vi "FeedbackDecode.vi"() -> ()   [LabVIEW 2020]
uses:
  FeedbackDecode_DecodeClust.ctl
  FeedbackDecode_MvntClust.ctl
  FeedbackDecode_EncodeClust.ctl
  FeedbackDecode_CogLoadClust.ctl
  <vilib>/Platform/TimedLoop/XDataNode/timing_clust.ctl
  <vilib>/Platform/TimedLoop/XDataNode/nitl_modes.ctl
  <vilib>/Platform/TimedLoop/XDataNode/wakeup.ctl
  <vilib>/DAQmx/write.llb/DAQmx Write (Analog DBL 1Chan 1Samp).vi
  subvi/FeedbackDecode_Globals.vi
  <vilib>/imath/engines/lvmath2/RunTimeEngine/BuiltInFunctions/reshapemx/NIMS_[GM]_reshapemx.vi
  <instcachedir>/0/NIMS_[GM]_reshapemx_98F4FEDA5D2741A4824CEDFB6097FB68.lvgen/NIMS_[GM]_reshapemx_98F4FEDA5D2741A4824CEDFB6097FB68_005.vi
  <vilib>/imath/engines/lvmath2/RunTimeEngine/BuiltInFunctions/rotate90/NIMS_rotate90.vi
  <instcachedir>/0/NIMS_rotate90_7DC1660D109944E092D2EB6E3185A1B6.lvgen/NIMS_rotate90_7DC1660D109944E092D2EB6E3185A1B6_005.vi
  <vilib>/imath/engines/lvmath2/RunTimeEngine/BuiltInFunctions/reshapemx/NIMS_[GV]_reshapemx.vi
  <instcachedir>/0/NIMS_[GV]_reshapemx_116A7F60707440F78CB0D64335A3F73C.lvgen/NIMS_[GV]_reshapemx_116A7F60707440F78CB0D64335A3F73C_001.vi
  <vilib>/imath/engines/lvmath2/RunTimeEngine/ErrorHandling/NIMS_Create Error From Enums.vi
  <vilib>/imath/engines/lvmath2/RunTimeEngine/NodeEndStatement/NIMS_NodeEndStatement_Output.vi
  <instcachedir>/0/NIMS_NodeEndStatement_Output_53EC0D466D134D7ABD903AC30B43404B.lvgen/NIMS_NodeEndStatement_Output_53EC0D466D134D7ABD903AC30B43404B_004.vi
  <vilib>/imath/engines/lvmath2/RunTimeEngine/ErrorHandling/NIMS_Finalize Error.vi
  subvi/FeedbackDecode_VariablesToString_Scalar.vi
  <vilib>/DAQmx/miscellaneous.llb/DAQmx Fill In Error Info.vi
  subvi/FeedbackDecode_VariablesToString_String.vi
  subvi/FeedbackDecode_VariablesToString_Array.vi
  <vilib>/Utility/file.llb/Read Delimited Spreadsheet (string).vi
  <vilib>/Utility/file.llb/Write Delimited Spreadsheet (string).vi
  <vilib>/platform/TimedLoop/XDataNode/XDataNode.xnode
  <vilib>/regexp/Match Regular Expression.xnode
  <vilib>/Platform/TimedLoop/XDataNode/XDNodeRunTimeDep.lvlib
  <resource>/objmgr/daqmx.rc
panel:
  out "ResourcesDir":path=path "Z:/Shared drives/CNI/Tasks/FeedbackDecode/resources"
  out "CurrMvnt":T1={"MvntMat"=[], "MvntName"="", "Tracking"=enum."False", "Radius"=0.15}
  in  "Exclude SE":bool
  out "DAQmx?":bool=TRUE
  out "NumComp":enum16{"1 Computer", "2 Computers"}(ring)
  out "BuildDir":path=path "/\"Z/Shared drives/CNI/Tasks/FeedbackDecode/build\""
  out "PupilTracker":bool
  out "CopySucc":bool
  out "Delete from D drive?":bool
  out "Copy to raid?":bool
  out "Don't save to database?":bool
  out "NextIdx":dbl
  in  "HeatMap Range":cluster{"Min":dbl, "Max":dbl}={"Min"=0.0, "Max"=50.0}
  out "RespRefArray":refnum<vi>[](array[refnum])
  out "VRELabel":T2(ring)
  out "StimTog":bool
  out "SelTog":bool
  out "StimCmd":string
  out "RespStr":string
  out "EvntReg":refnum<event-registration>
  out "MvntEvnt":refnum<user-event>
  out "DataDir":path=path "D:/FeedbackDecode"
  out "PulseStim":bool
  out "BaseCnt3":i64=-9223372036854775808
  out "NIPTime":dbl
  out "ParamsTableLoc":cluster{"Left":i32, "Width":u32}={"Left"=1206, "Width"=743}
  out "iTiming":T3={"Dur"={"ASD"=1000.0, "ARD"=5000.0, "ART"=5000.0, "ETD"=500.0}, "Rnd"={"ASDR"=0.0, "ARDR"=0.0, "ARTR"=0.0, "ETDR"=0.0}, "Act"={"ASDA"=0.0, "ARDA"=0.0, "ARTA"=0.0, "ETDA"=0.0}}
  in  "LVTab":T4(tab)
  out "TrainCnt":dbl
  in  "DecodeClust":T5={"TrainParams"={"Lag"=0.0, "KernelWidth"=0.3, "TargRad"=0.15}, "Kinematics"={"Thumb"=0.0, "Index"=0.0, "Middle"=0.0, "Ring"=0.0, "Little"=0.0, "ThumbInt"=0.0, "IndexInt"=0.0, "RingInt"=0.0, "LittleInt"=0.0, "Wrist"=0.0, "WristYaw"=0.0, "WristRoll"=0.0}, "CtrlButtons"={"AcqTraining"=FALSE, "ApplyBaseline"=FALSE, "ApplyTraining"=FALSE, "LoadTrainFile"=FALSE, "CAR"=FALSE, "NIPSpikes"=FALSE, "AcqBaseline"=FALSE, "Stop"=FALSE, "ResetTrial"=FALSE, "CalDEKA"=FALSE, "HideSphrs"=FALSE, "StartTrials"=FALSE, "AutoPop"=FALSE, "ResetVRE"=FALSE, "StopVRE"=FALSE, "AcqCAR"=FALSE, "ConARD"=FALSE, "DEKARestart"=FALSE, "ConnDEKA"=FALSE}, "CompID"={"LV"={"Name"="PNILABVIEW", "IP"="127.0.0.1"}, "ML"={"Name"="PNIMATLAB", "IP"="127.0.0.2"}}, "KMvntClust"={"KGain"=[[1.0, 1.0, -1.0, 1.0], [1.0, 1.0, -1.0, 1.0], [1.0, 1.0, -1.0, 1.0], [1.0, 1.0, -1.0, 1.0], [1.0, 1.0, -1.0, 1.0], [1.0, 1.0, -1.0, 1.0], [1.0, 1.0, -1.0, 1.0], [1.0, 1.0, -1.0, 1.0], [1.0, 1.0, -1.0, 1.0], [1.0, 1.0, -1.0, 1.0], [1.0, 1.0, -1.0, 1.0], [1.0, 1.0, -1.0, 1.0]], "KMvnts"={"Thumb"=TRUE, "Index"=TRUE, "Middle"=TRUE, "Ring"=TRUE, "Little"=TRUE, "ThumbInt"=TRUE, "IndexInt"=TRUE, "RingInt"=TRUE, "LittleInt"=TRUE, "WristPitch"=TRUE, "WristYaw"=TRUE, "WristRoll"=TRUE}, "KThresh"=[[0.2, 0.2, -1.0, 1.0], [0.2, 0.2, -1.0, 1.0], [0.2, 0.2, -1.0, 1.0], [0.2, 0.2, -1.0, 1.0], [0.2, 0.2, -1.0, 1.0], [0.2, 0.2, -1.0, 1.0], [0.2, 0.2, -1.0, 1.0], [0.2, 0.2, -1.0, 1.0], [0.2, 0.2, -1.0, 1.0], [0.2, 0.2, -1.0, 1.0], [0.2, 0.2, -1.0, 1.0], [0.2, 0.2, -1.0, 1.0]], "CtrlMode"=[enum."Position", enum."Position", enum."Position", enum."Position", enum."Position", enum."Position", enum."Position", enum."Position", enum."Position", enum."Position", enum."Position", enum."Position"], "CtrlSpd"=[1.0, 1.0, 1.0, 1.0, 1.0, 1.0, 1.0, 1.0, 1.0, 1.0, 1.0, 1.0]}, "ClearUEA"=FALSE, "Targets"={"Thumb"=0.0, "Index"=0.0, "Middle"=0.0, "Ring"=0.0, "Little"=0.0, "ThumbInt"=0.0, "IndexInt"=0.0, "RingInt"=0.0, "LittleInt"=0.0, "Wrist"=0.0, "WristYaw"=0.0, "WristRoll"=0.0}, "KUEAArray"=[{"Boolean 1"=FALSE, "Boolean 2"=FALSE, "Boolean 3"=FALSE, "Boolean 4"=FALSE, "Boolean 5"=FALSE, "Boolean 6"=FALSE, "Boolean 7"=FALSE, "Boolean 8"=FALSE, "Boolean 9"=FALSE, "Boolean 10"=FALSE, "Boolean 11"=FALSE, "Boolean 12"=FALSE, "Boolean 13"=FALSE, "Boolean 14"=FALSE, "Boolean 15"=FALSE, "Boolean 16"=FALSE, "Boolean 17"=FALSE, "Boolean 18"=FALSE, "Boolean 19"=FALSE, "Boolean 20"=FALSE, "Boolean 21"=FALSE, "Boolean 22"=FALSE, "Boolean 23"=FALSE, "Boolean 24"=FALSE, "Boolean 25"=FALSE, "Boolean 26"=FALSE, "Boolean 27"=FALSE, "Boolean 28"=FALSE, "Boolean 29"=FALSE, "Boolean 30"=FALSE, "Boolean 31"=FALSE, "Boolean 32"=FALSE, "Boolean 33"=FALSE, "Boolean 34"=FALSE, "Boolean 35"=FALSE, "Boolean 36"=FALSE, "Boolean 37"=FALSE, "Boolean 38"=FALSE, "Boolean 39"=FALSE, "Boolean 40"=FALSE, "Boolean 41"=FALSE, "Boolean 42"=FALSE, "Boolean 43"=FALSE, "Boolean 44"=FALSE, "Boolean 45"=FALSE, "Boolean 46"=FALSE, "Boolean 47"=FALSE, "Boolean 48"=FALSE, "Boolean 49"=FALSE, "Boolean 50"=FALSE, "Boolean 51"=FALSE, "Boolean 52"=FALSE, "Boolean 53"=FALSE, "Boolean 54"=FALSE, "Boolean 55"=FALSE, "Boolean 56"=FALSE, "Boolean 57"=FALSE, "Boolean 58"=FALSE, "Boolean 59"=FALSE, "Boolean 60"=FALSE, "Boolean 61"=FALSE, "Boolean 62"=FALSE, "Boolean 63"=FALSE, "Boolean 64"=FALSE, "Boolean 65"=FALSE, "Boolean 66"=FALSE, "Boolean 67"=FALSE, "Boolean 68"=FALSE, "Boolean 69"=FALSE, "Boolean 70"=FALSE, "Boolean 71"=FALSE, "Boolean 72"=FALSE, "Boolean 73"=FALSE, "Boolean 74"=FALSE, "Boolean 75"=FALSE, "Boolean 76"=FALSE, "Boolean 77"=FALSE, "Boolean 78"=FALSE, "Boolean 79"=FALSE, "Boolean 80"=FALSE, "Boolean 81"=FALSE, "Boolean 82"=FALSE, "Boolean 83"=FALSE, "Boolean 84"=FALSE, "Boolean 85"=FALSE, "Boolean 86"=FALSE, "Boolean 87"=FALSE, "Boolean 88"=FALSE, "Boolean 89"=FALSE, "Boolean 90"=FALSE, "Boolean 91"=FALSE, "Boolean 92"=FALSE, "Boolean 93"=FALSE, "Boolean 94"=FALSE, "Boolean 95"=FALSE, "Boolean 96"=FALSE, "Boolean 97"=FALSE, "Boolean 98"=FALSE, "Boolean 99"=FALSE, "Boolean 100"=FALSE}, {"Boolean 1"=FALSE, "Boolean 2"=FALSE, "Boolean 3"=FALSE, "Boolean 4"=FALSE, "Boolean 5"=FALSE, "Boolean 6"=FALSE, "Boolean 7"=FALSE, "Boolean 8"=FALSE, "Boolean 9"=FALSE, "Boolean 10"=FALSE, "Boolean 11"=FALSE, "Boolean 12"=FALSE, "Boolean 13"=FALSE, "Boolean 14"=FALSE, "Boolean 15"=FALSE, "Boolean 16"=FALSE, "Boolean 17"=FALSE, "Boolean 18"=FALSE, "Boolean 19"=FALSE, "Boolean 20"=FALSE, "Boolean 21"=FALSE, "Boolean 22"=FALSE, "Boolean 23"=FALSE, "Boolean 24"=FALSE, "Boolean 25"=FALSE, "Boolean 26"=FALSE, "Boolean 27"=FALSE, "Boolean 28"=FALSE, "Boolean 29"=FALSE, "Boolean 30"=FALSE, "Boolean 31"=FALSE, "Boolean 32"=FALSE, "Boolean 33"=FALSE, "Boolean 34"=FALSE, "Boolean 35"=FALSE, "Boolean 36"=FALSE, "Boolean 37"=FALSE, "Boolean 38"=FALSE, "Boolean 39"=FALSE, "Boolean 40"=FALSE, "Boolean 41"=FALSE, "Boolean 42"=FALSE, "Boolean 43"=FALSE, "Boolean 44"=FALSE, "Boolean 45"=FALSE, "Boolean 46"=FALSE, "Boolean 47"=FALSE, "Boolean 48"=FALSE, "Boolean 49"=FALSE, "Boolean 50"=FALSE, "Boolean 51"=FALSE, "Boolean 52"=FALSE, "Boolean 53"=FALSE, "Boolean 54"=FALSE, "Boolean 55"=FALSE, "Boolean 56"=FALSE, "Boolean 57"=FALSE, "Boolean 58"=FALSE, "Boolean 59"=FALSE, "Boolean 60"=FALSE, "Boolean 61"=FALSE, "Boolean 62"=FALSE, "Boolean 63"=FALSE, "Boolean 64"=FALSE, "Boolean 65"=FALSE, "Boolean 66"=FALSE, "Boolean 67"=FALSE, "Boolean 68"=FALSE, "Boolean 69"=FALSE, "Boolean 70"=FALSE, "Boolean 71"=FALSE, "Boolean 72"=FALSE, "Boolean 73"=FALSE, "Boolean 74"=FALSE, "Boolean 75"=FALSE, "Boolean 76"=FALSE, "Boolean 77"=FALSE, "Boolean 78"=FALSE, "Boolean 79"=FALSE, "Boolean 80"=FALSE, "Boolean 81"=FALSE, "Boolean 82"=FALSE, "Boolean 83"=FALSE, "Boolean 84"=FALSE, "Boolean 85"=FALSE, "Boolean 86"=FALSE, "Boolean 87"=FALSE, "Boolean 88"=FALSE, "Boolean 89"=FALSE, "Boolean 90"=FALSE, "Boolean 91"=FALSE, "Boolean 92"=FALSE, "Boolean 93"=FALSE, "Boolean 94"=FALSE, "Boolean 95"=FALSE, "Boolean 96"=FALSE, "Boolean 97"=FALSE, "Boolean 98"=FALSE, "Boolean 99"=FALSE, "Boolean 100"=FALSE}], "ReTrain"=FALSE, "TargDist"=[0.0, 0.0, 0.0, 0.0, 0.0, 0.0], "State"=enum."Initialize", "KalmanType"=enum."Mean", "EventStr"="SS.KalmanElects=[];SS.KalmanMvnts=[1,2,3,4,5,6,7,8,9,10,11,12];SS.KalmanGain=[1.0,1.0;1.0,1.0;1.0,1.0;1.0,1.0;1.0,1.0;1.0,1.0;1.0,1.0;1.0,1.0;1.0,1.0;1.0,1.0;1.0,1.0;1.0,1.0;];SS.KalmanThresh=[0.2,0.2;0.2,0.2;0.2,0.2;0.2,0.2;0.2,0.2;0.2,0.2;0.2,0.2;0.2,0.2;0.2,0.2;0.2,0.2;0.2,0.2;0.2,0.2;];SS.CtrlMode={'Position','Position','Position','Position','Position','Position','Position','Position','Position','Position','Position','Position'};SS.CtrlSpeed=[1.0,1.0,1.0,1.0,1.0,1.0,1.0,1.0,1.0,1.0,1.0,1.0];SS.Lag=0.00;SS.KernelWidth=0.30;SS.TargRad=0.15;SS.DataFolder='20210325-092059';SS.DataDir='D@\\FeedbackDecode';SS.BuildDir='Z@\\Shared drives\\CNI\\Tasks\\FeedbackDecode\\build';SS.BadUEAElects=[];SS.SelElect=0;SS.ThreshMode='RMS Auto';SS.ThreshVal=-5.00;SS.AcqTraining=0;SS.ApplyBaseline=0;SS.ApplyTraining=0;SS.LoadTrainFile=0;SS.CAR=0;SS.NIPSpikes=0;SS.AcqBaseline=0;SS.Stop=0;SS.ResetTrial=0;SS.CalibrateDEKA=0;SS.HideSpheres=0;SS.StartTrials=0;SS.AutoPop=0;SS.ResetVRE=0;SS.StopVRE=0;SS.AcqCAR=0;SS.ConnectARD=0;SS.RestartDEKA=0;SS.ConnectDEKA=0;SS.KalmanType='Mean';SS.ReTrain=0;SS.KalmanEMG=[];SS.KinSrc='Off';SS.AllPairs=1;SS.AutoThresh=0.40;SS.KEMGExtra=[];SS.BadEMGChans=[];SS.LinkedDOF={};SS.AutoPopType=2;SS.CARType='Standard';SS.Map='pNeural/pEMG';SS.TestType='MSMS';SS.ResetVRE=0;SS.StartMLAux=1;SS.StartXippRec=1;SS.Log10=0;SS.LimitExt=0;SS.DynFlag=0;SS.Prosthesis='MaleRight';SS.FreeParam=1.00000;SS.GoalNoise=0.00000;SS.NumComp='1 Computer';SS.StartARD=0;SS.StartTaska=0;SS.StartTaskaSens=0;SS.EnableTrigger=0;SS.EEGTrigger=0;SS.ConnectECG=0;SS.ECGTriggerTargets=0;SS.SecondaryTask=0;SS.SecondaryTaskMinBetweenStim=3000.00000;SS.SecondaryTaskVarBetweenStim=2000.00000;SS.SecondaryTaskStimDur=1000.00000;SS.RecordIMUwithTraining=0;SS.ConnectIMU=0;SS.StimCell={};SS.StimMode='Off';SS.StimStepSize=[1.00,1.00,0.00];SS.ManualStim=0;SS.Jitter=0;SS.BFreq=0;SS.BAmp=0;", "SelElect"=0.0, "KinSrc"=enum."Off", "HoverElect"=1.0, "RasterWin"=15.0, "WfCnt"=50.0, "ClearWfs"=FALSE, "ApplyThresh"=FALSE, "ThreshVal"=-5.0, "ThreshMode"=enum."RMS Auto", "DataFolder"="20210325-092059", "ClearEMG"=FALSE, "KEMGClust"={"Boolean 92"=FALSE, "Boolean 82"=FALSE, "Boolean 72"=FALSE, "Boolean 62"=FALSE, "Boolean 52"=FALSE, "Boolean 42"=FALSE, "Boolean 32"=FALSE, "Boolean 22"=FALSE, "Boolean 12"=FALSE, "Boolean 2"=FALSE, "Boolean 93"=FALSE, "Boolean 83"=FALSE, "Boolean 73"=FALSE, "Boolean 63"=FALSE, "Boolean 53"=FALSE, "Boolean 43"=FALSE, "Boolean 33"=FALSE, "Boolean 23"=FALSE, "Boolean 13"=FALSE, "Boolean 3"=FALSE, "Boolean 94"=FALSE, "Boolean 84"=FALSE, "Boolean 74"=FALSE, "Boolean 64"=FALSE, "Boolean 54"=FALSE, "Boolean 44"=FALSE, "Boolean 34"=FALSE, "Boolean 24"=FALSE, "Boolean 14"=FALSE, "Boolean 4"=FALSE, "Boolean 95"=FALSE, "Boolean 85"=FALSE, "Boolean 75"=FALSE, "Boolean 65"=FALSE, "Boolean 55"=FALSE, "Boolean 45"=FALSE, "Boolean 35"=FALSE, "Boolean 25"=FALSE, "Boolean 15"=FALSE, "Boolean 5"=FALSE, "Boolean 96"=FALSE, "Boolean 86"=FALSE, "Boolean 76"=FALSE, "Boolean 66"=FALSE, "Boolean 56"=FALSE, "Boolean 46"=FALSE, "Boolean 36"=FALSE, "Boolean 26"=FALSE, "Boolean 16"=FALSE, "Boolean 6"=FALSE, "Boolean 97"=FALSE, "Boolean 87"=FALSE, "Boolean 77"=FALSE, "Boolean 67"=FALSE, "Boolean 57"=FALSE, "Boolean 47"=FALSE, "Boolean 37"=FALSE, "Boolean 27"=FALSE, "Boolean 17"=FALSE, "Boolean 7"=FALSE, "Boolean 98"=FALSE, "Boolean 88"=FALSE, "Boolean 78"=FALSE, "Boolean 68"=FALSE, "Boolean 58"=FALSE, "Boolean 48"=FALSE, "Boolean 38"=FALSE, "Boolean 28"=FALSE, "Boolean 18"=FALSE, "Boolean 8"=FALSE, "Boolean 99"=FALSE, "Boolean 89"=FALSE, "Boolean 79"=FALSE, "Boolean 69"=FALSE, "Boolean 59"=FALSE, "Boolean 49"=FALSE, "Boolean 39"=FALSE, "Boolean 29"=FALSE, "Boolean 19"=FALSE, "Boolean 9"=FALSE}, "EvntFlag"=FALSE, "FillUEA"=FALSE, "FillEMG"=FALSE, "FillMvnts"=FALSE, "BadUEAElects"=[], "KEMGExtra"=[], "AllPairs"=TRUE, "AutoThresh"=0.4, "BadEMGChans"=[], "LinkedDOF"="{}", "AutoPopType"=enum."Gram", "CARType"=enum."Standard", "*Map"=enum."N2021/pEMG", "GainFill"=1.0, "ThreshFill"=0.2, "TestType"=enum."MSMS", "Outcome"=enum."---", "TrialCnt"=[[0.0, 0.0, 0.0, 0.0, 0.0, 0.0, 0.0, 0.0, 0.0, 0.0, 0.0, 0.0], [0.0, 0.0, 0.0, 0.0, 0.0, 0.0, 0.0, 0.0, 0.0, 0.0, 0.0, 0.0]], "ClearTrials"=FALSE, "Log10"=FALSE, "KDFFile"="", "LimitExt"=FALSE, "*Prosthesis"=enum."MaleRight", "StartML"=TRUE, "StartMLAux"=TRUE, "StartRec"=TRUE, "DynaThr"=FALSE, "ModeFill"=enum."Position", "SpdFill"=1.0, "DEKAMode"=enum."Position", "FreeParam"=1.0, "GoalNoise"=0.0, "Load NN"=FALSE, "ExportTrain"=FALSE, "NumComp"=enum."1 Computer", "DataDir"="D@\\FeedbackDecode", "BuildDir"="Z@\\Shared drives\\CNI\\Tasks\\FeedbackDecode\\build", "LatchingFilter"=FALSE, "Trigger"=FALSE, "StartARD"=FALSE, "StartTaska"=FALSE, "StartTaskaSens"=FALSE} {"SpdFill" min=0.0 max=10.0 step=0.1; "RasterWin" min=1.0 max=30.0 step=1.0; "ThreshFill" min=0.0 max=10.0 step=0.01; "GainFill" min=0.0 max=10.0 step=0.1; "AutoThresh" min=0.0 max=1.0; "Targets"."LittleInt" min=0.0 max=1.0 step=0.01; "Targets"."WristRoll" min=0.0 max=1.0 step=0.01; "Targets"."WristYaw" min=0.0 max=1.0 step=0.01; "Targets"."Wrist" min=0.0 max=1.0 step=0.01; "Targets"."Little" min=0.0 max=1.0 step=0.01; "Targets"."Thumb" min=0.0 max=1.0 step=0.01; "Targets"."RingInt" min=0.0 max=1.0 step=0.01; "Targets"."IndexInt" min=0.0 max=1.0 step=0.01; "Targets"."ThumbInt" min=0.0 max=1.0 step=0.01; "Targets"."Ring" min=0.0 max=1.0 step=0.01; "Targets"."Middle" min=0.0 max=1.0 step=0.01; "Targets"."Index" min=0.0 max=1.0 step=0.01; "KMvntClust"."CtrlSpd" min=0 max=10; "KMvntClust"."KThresh" min=0 max=1; "KMvntClust"."KGain" min=0; "Kinematics"."LittleInt" min=0.0 max=1.0 step=0.01; "Kinematics"."WristRoll" min=0.0 max=1.0 step=0.01; "Kinematics"."WristYaw" min=0.0 max=1.0 step=0.01; "Kinematics"."Wrist" min=0.0 max=1.0 step=0.01; "Kinematics"."Little" min=0.0 max=1.0 step=0.01; "Kinematics"."Thumb" min=0.0 max=1.0 step=0.01; "Kinematics"."RingInt" min=0.0 max=1.0 step=0.01; "Kinematics"."IndexInt" min=0.0 max=1.0 step=0.01; "Kinematics"."ThumbInt" min=0.0 max=1.0 step=0.01; "Kinematics"."Ring" min=0.0 max=1.0 step=0.01; "Kinematics"."Middle" min=0.0 max=1.0 step=0.01; "Kinematics"."Index" min=0.0 max=1.0 step=0.01; "TrainParams"."TargRad" step=0.05 format="%#.2g"; "TrainParams"."KernelWidth" step=0.05 format="%#.2g"}
  in  "Timing":T3={"Dur"={"ASD"=1000.0, "ARD"=5000.0, "ART"=5000.0, "ETD"=500.0}, "Rnd"={"ASDR"=0.0, "ARDR"=0.0, "ARTR"=0.0, "ETDR"=0.0}, "Act"={"ASDA"=0.0, "ARDA"=0.0, "ARTA"=0.0, "ETDA"=0.0}}
  in  "MvntBuilder":T6={"MvntType"={"Thumb"=enum."False", "Index"=enum."False", "Middle"=enum."False", "Ring"=enum."False", "Little"=enum."False", "ThumbInt"=enum."False", "IndexInt"=enum."False", "RingInt"=enum."False", "LittleInt"=enum."False", "WristPitch"=enum."False", "WristYaw"=enum."False", "WristRoll"=enum."False"}, "MvntParams"={"Amp"=1.0, "Delay"=0.0, "Rise"=0.7, "Hold"=3.0}, "MvntList"=[{"MvntMat"=[[0.0, 0.0, 0.0, 0.0], [0.0, 0.0, 0.0, 0.0], [0.0, 0.0, 0.0, 0.0], [0.0, 0.0, 0.0, 0.0], [0.0, 0.0, 0.0, 0.0], [0.0, 0.0, 0.0, 0.0], [0.0, 0.0, 0.0, 0.0], [0.0, 0.0, 0.0, 0.0], [0.0, 0.0, 0.0, 0.0], [0.0, 0.0, 0.0, 0.0], [0.0, 0.0, 0.0, 0.0], [0.0, 0.0, 0.0, 0.0]], "MvntName"="", "Tracking"=enum."False", "Radius"=0.15}], "Set"=FALSE, "Clear"=FALSE, "Load"=FALSE, "Mode"=enum."Block", "NTrials"=10.0, "TargParams"={"Gain"=1.0, "Radius"=0.15, "Acc"=0.8}, "Save"=FALSE, "PercTrials"=0.1} {"PercTrials" format="%#_2g"; "NTrials" min=1.0 max=100.0 step=1.0; "MvntList"."Radius" min=0.0 max=1.0 step=0.01; "TargParams"."Acc" min=0.0 max=1.0 step=0.01; "TargParams"."Radius" min=0.0 max=1.0 step=0.01; "TargParams"."Gain" min=-1.0 max=1.0 step=0.01; "MvntParams"."Hold" min=0.0 step=0.1; "MvntParams"."Rise" min=0.0 step=0.1; "MvntParams"."Delay" min=0.0 step=0.1; "MvntParams"."Amp" min=-1.0 max=1.0 step=0.1}
  in  "ManualClust":T7 {"WristRoll" scale=-1.0..1.0; "WristYaw" scale=-1.0..1.0; "WristPitch" scale=-1.0..1.0; "LittleInt" scale=-1.0..1.0; "RingInt" scale=-1.0..1.0; "IndexInt" scale=-1.0..1.0; "ThumbInt" scale=-1.0..1.0; "Little" scale=-1.0..1.0; "Ring" scale=-1.0..1.0; "Middle" scale=-1.0..1.0; "Index" scale=-1.0..1.0; "Thumb" scale=-1.0..1.0}
  in  "ManualDOF":T8
  in  "EncodeClust":T9={"ParamsTable"=[], "Sel"=[], "Stim"=FALSE, "StimMode"=enum."Off", "StimStep"=[enum."1uA", enum."1uA", enum."Off"], "Jitter"=FALSE, "Pulse"=FALSE, "BFreq"=0.0, "BAmp"=0.0, "UEAArray"=[{"Boolean 1"=FALSE, "Boolean 2"=FALSE, "Boolean 3"=FALSE, "Boolean 4"=FALSE, "Boolean 5"=FALSE, "Boolean 6"=FALSE, "Boolean 7"=FALSE, "Boolean 8"=FALSE, "Boolean 9"=FALSE, "Boolean 10"=FALSE, "Boolean 11"=FALSE, "Boolean 12"=FALSE, "Boolean 13"=FALSE, "Boolean 14"=FALSE, "Boolean 15"=FALSE, "Boolean 16"=FALSE, "Boolean 17"=FALSE, "Boolean 18"=FALSE, "Boolean 19"=FALSE, "Boolean 20"=FALSE, "Boolean 21"=FALSE, "Boolean 22"=FALSE, "Boolean 23"=FALSE, "Boolean 24"=FALSE, "Boolean 25"=FALSE, "Boolean 26"=FALSE, "Boolean 27"=FALSE, "Boolean 28"=FALSE, "Boolean 29"=FALSE, "Boolean 30"=FALSE, "Boolean 31"=FALSE, "Boolean 32"=FALSE, "Boolean 33"=FALSE, "Boolean 34"=FALSE, "Boolean 35"=FALSE, "Boolean 36"=FALSE, "Boolean 37"=FALSE, "Boolean 38"=FALSE, "Boolean 39"=FALSE, "Boolean 40"=FALSE, "Boolean 41"=FALSE, "Boolean 42"=FALSE, "Boolean 43"=FALSE, "Boolean 44"=FALSE, "Boolean 45"=FALSE, "Boolean 46"=FALSE, "Boolean 47"=FALSE, "Boolean 48"=FALSE, "Boolean 49"=FALSE, "Boolean 50"=FALSE, "Boolean 51"=FALSE, "Boolean 52"=FALSE, "Boolean 53"=FALSE, "Boolean 54"=FALSE, "Boolean 55"=FALSE, "Boolean 56"=FALSE, "Boolean 57"=FALSE, "Boolean 58"=FALSE, "Boolean 59"=FALSE, "Boolean 60"=FALSE, "Boolean 61"=FALSE, "Boolean 62"=FALSE, "Boolean 63"=FALSE, "Boolean 64"=FALSE, "Boolean 65"=FALSE, "Boolean 66"=FALSE, "Boolean 67"=FALSE, "Boolean 68"=FALSE, "Boolean 69"=FALSE, "Boolean 70"=FALSE, "Boolean 71"=FALSE, "Boolean 72"=FALSE, "Boolean 73"=FALSE, "Boolean 74"=FALSE, "Boolean 75"=FALSE, "Boolean 76"=FALSE, "Boolean 77"=FALSE, "Boolean 78"=FALSE, "Boolean 79"=FALSE, "Boolean 80"=FALSE, "Boolean 81"=FALSE, "Boolean 82"=FALSE, "Boolean 83"=FALSE, "Boolean 84"=FALSE, "Boolean 85"=FALSE, "Boolean 86"=FALSE, "Boolean 87"=FALSE, "Boolean 88"=FALSE, "Boolean 89"=FALSE, "Boolean 90"=FALSE, "Boolean 91"=FALSE, "Boolean 92"=FALSE, "Boolean 93"=FALSE, "Boolean 94"=FALSE, "Boolean 95"=FALSE, "Boolean 96"=FALSE, "Boolean 97"=FALSE, "Boolean 98"=FALSE, "Boolean 99"=FALSE, "Boolean 100"=FALSE}, {"Boolean 1"=FALSE, "Boolean 2"=FALSE, "Boolean 3"=FALSE, "Boolean 4"=FALSE, "Boolean 5"=FALSE, "Boolean 6"=FALSE, "Boolean 7"=FALSE, "Boolean 8"=FALSE, "Boolean 9"=FALSE, "Boolean 10"=FALSE, "Boolean 11"=FALSE, "Boolean 12"=FALSE, "Boolean 13"=FALSE, "Boolean 14"=FALSE, "Boolean 15"=FALSE, "Boolean 16"=FALSE, "Boolean 17"=FALSE, "Boolean 18"=FALSE, "Boolean 19"=FALSE, "Boolean 20"=FALSE, "Boolean 21"=FALSE, "Boolean 22"=FALSE, "Boolean 23"=FALSE, "Boolean 24"=FALSE, "Boolean 25"=FALSE, "Boolean 26"=FALSE, "Boolean 27"=FALSE, "Boolean 28"=FALSE, "Boolean 29"=FALSE, "Boolean 30"=FALSE, "Boolean 31"=FALSE, "Boolean 32"=FALSE, "Boolean 33"=FALSE, "Boolean 34"=FALSE, "Boolean 35"=FALSE, "Boolean 36"=FALSE, "Boolean 37"=FALSE, "Boolean 38"=FALSE, "Boolean 39"=FALSE, "Boolean 40"=FALSE, "Boolean 41"=FALSE, "Boolean 42"=FALSE, "Boolean 43"=FALSE, "Boolean 44"=FALSE, "Boolean 45"=FALSE, "Boolean 46"=FALSE, "Boolean 47"=FALSE, "Boolean 48"=FALSE, "Boolean 49"=FALSE, "Boolean 50"=FALSE, "Boolean 51"=FALSE, "Boolean 52"=FALSE, "Boolean 53"=FALSE, "Boolean 54"=FALSE, "Boolean 55"=FALSE, "Boolean 56"=FALSE, "Boolean 57"=FALSE, "Boolean 58"=FALSE, "Boolean 59"=FALSE, "Boolean 60"=FALSE, "Boolean 61"=FALSE, "Boolean 62"=FALSE, "Boolean 63"=FALSE, "Boolean 64"=FALSE, "Boolean 65"=FALSE, "Boolean 66"=FALSE, "Boolean 67"=FALSE, "Boolean 68"=FALSE, "Boolean 69"=FALSE, "Boolean 70"=FALSE, "Boolean 71"=FALSE, "Boolean 72"=FALSE, "Boolean 73"=FALSE, "Boolean 74"=FALSE, "Boolean 75"=FALSE, "Boolean 76"=FALSE, "Boolean 77"=FALSE, "Boolean 78"=FALSE, "Boolean 79"=FALSE, "Boolean 80"=FALSE, "Boolean 81"=FALSE, "Boolean 82"=FALSE, "Boolean 83"=FALSE, "Boolean 84"=FALSE, "Boolean 85"=FALSE, "Boolean 86"=FALSE, "Boolean 87"=FALSE, "Boolean 88"=FALSE, "Boolean 89"=FALSE, "Boolean 90"=FALSE, "Boolean 91"=FALSE, "Boolean 92"=FALSE, "Boolean 93"=FALSE, "Boolean 94"=FALSE, "Boolean 95"=FALSE, "Boolean 96"=FALSE, "Boolean 97"=FALSE, "Boolean 98"=FALSE, "Boolean 99"=FALSE, "Boolean 100"=FALSE}], "AdjClust"={"Add"=FALSE, "Sub"=FALSE, "Val"=[1.0, 100.0, 10.0, 500.0, 0.2], "B"=[FALSE, FALSE, FALSE, FALSE, FALSE], "Inc+"=["x+1", "x+1", "x+10", "x+10", "x+0.1"], "Set"=FALSE, "LoadTable"=FALSE, "SaveTable"=FALSE, "ClearTable"=FALSE, "DeleteSel"=FALSE, "Inc-"=["x-1", "x-1", "x-10", "x-10", "x-0.1"]}, "PresetTable"=[], "SelPreset"=[], "SortClust"={"Region"=FALSE, "Receptor"=FALSE, "Electrode"=FALSE, "Min Amp"=FALSE, "Max Amp"=FALSE, "Min Freq"=FALSE, "Max Freq"=FALSE, "Duration"=FALSE}, "SelSort"={"Sel"=FALSE}, "PresetClust"={"Load"=FALSE, "Clear"=FALSE, "Save"=FALSE, "Del"=FALSE}, "RespClust"={"RespType"=enum."Sensor Map", "OpenResp"=FALSE}, "AmpLimit"=100.0, "FreqLimit"=500.0, "DurLimit"=0.2, "Wait Period"=0.5, "Train Period"=0.5, "ManualType"=enum."Max"} {"Train Period" min=0.0 max=100.0 step=0.1; "Wait Period" min=0.0 max=100.0 step=0.1; "DurLimit" min=0.0 max=1.0 step=0.01; "FreqLimit" min=0.0 max=500.0 step=1.0; "AmpLimit" min=0.0 max=100.0 step=1.0; "BAmp" min=0.0 max=100.0 step=1.0; "BFreq" min=0.0 max=100.0 step=1.0}
  in  "Sensor Tab Control":enum32{"DEKA", "Analog", "TASKA"}(tab)
  out "DekaSensors":waveform(dbl)[](graph)
  out "StimWfGraph":dbl[](graph)
  in  "Stim Thresholds":dbl[](array[numeric])=[0.0, 0.0, 0.0, 0.0, 0.0, 0.0, 0.0, 0.0, 0.0, 0.0, 0.0, 0.0, 0.0]
  in  "DekaSensorBreakThreshold":dbl[](array[numeric])=[40.0, 40.0, 40.0, 40.0, 40.0, 40.0, 40.0, 40.0, 40.0, 40.0, 40.0, 40.0, 40.0]
  out "AnlgPlot":waveform(dbl)[](graph)=[{"t0"=timestamp(27834 s since 1904-01-01), "dt"=1.0, "Y"=[2.75375102500714]}, {"t0"=timestamp(27834 s since 1904-01-01), "dt"=1.0, "Y"=[2.3160330296785294]}, {"t0"=timestamp(27834 s since 1904-01-01), "dt"=1.0, "Y"=[1.270290647354958]}, {"t0"=timestamp(27834 s since 1904-01-01), "dt"=1.0, "Y"=[1.3014283460420921]}]
  in  "OffSet":dbl
  in  "LoadCyberGlove":bool
  in  "TASKARestPositions":string="Rest Positions"
  in  "ThumbIntSet":dbl caption="ThumbInt" min=0.0 max=1.0
  in  "ThumbSet":dbl caption="Thumb" min=0.0 max=1.0
  in  "PinkySet":dbl caption="Pinky" min=0.0 max=1.0
  in  "RingSet":dbl caption="Ring" min=0.0 max=1.0
  in  "MiddleSet":dbl caption="Middle" min=0.0 max=1.0
  in  "IndexSet":dbl caption="Index" min=0.0 max=1.0
  in  "CalibrateTASKA":bool
  in  "Beta Mode":string(combo)="Fixed"
  in  "Computer Goal":string(combo)="Close"
  out "TASKA Pressure":waveform(dbl)[](graph)=[{"t0"=timestamp(87262 s since 1904-01-01), "dt"=1.0, "Y"=[0.0]}, {"t0"=timestamp(87262 s since 1904-01-01), "dt"=1.0, "Y"=[0.0]}, {"t0"=timestamp(87262 s since 1904-01-01), "dt"=1.0, "Y"=[0.0]}]
  out "TASKA IR":waveform(dbl)[](graph)=[{"t0"=timestamp(87262 s since 1904-01-01), "dt"=1.0, "Y"=[4.0]}, {"t0"=timestamp(87262 s since 1904-01-01), "dt"=1.0, "Y"=[0.0]}, {"t0"=timestamp(87262 s since 1904-01-01), "dt"=1.0, "Y"=[0.0]}]
  in  "TASKA Shared Control":bool
  in  "TASKASharedControlBeta":dbl caption="Beta" min=0.0 max=1.0
  in  "ThumbShare":bool
  in  "IndexShare":bool
  in  "RingShare":bool
  in  "MiddleShare":bool
  in  "Reset Calibration":bool
  in  "TASKASharedControlIncrememnt":dbl caption="Inc." min=0.0 max=1.0
  in  "TASKA Timer":bool
  in  "TASKA Reset Break":bool
  in  "TASKA Reset Success":bool
  out "WAVChart":dbl[](graph)=[0.01885986328125, 0.02471923828125, 0.026458740234375, 0.019622802734375, 0.015625, 0.016571044921875, 0.017852783203125, 0.016937255859375, 0.02349853515625, 0.0262451171875, 0.021697998046875, 0.01995849609375, 0.013427734375, 0.008819580078125, 0.013916015625, 0.016693115234375, 0.0172119140625, 0.023468017578125, 0.0235595703125, 0.018890380859375, 0.022369384765625, 0.022003173828125, 0.019378662109375, 0.017578125, 0.0115966796875, 0.011688232421875, 0.011016845703125, 0.007659912109375, 0.012359619140625, 0.015167236328125, 0.010162353515625, 0.00787353515625, 0.010009765625, 0.01434326171875, 0.018524169921875, 0.019012451171875, 0.019317626953125, 0.019500732421875, 0.021514892578125, 0.021514892578125, 0.0233154296875, 0.02276611328125, 0.0174560546875, 0.018585205078125, 0.019439697265625, 0.01959228515625, 0.0185546875, 0.015594482421875, 0.01593017578125, 0.0162353515625, 0.013427734375, 0.01519775390625, 0.005340576171875, 0.008026123046875, 0.00811767578125, 0.004669189453125, 0.008148193359375, 0.00384521484375, 0.007598876953125, 0.007354736328125, 0.009735107421875, 0.01580810546875, 0.01385498046875, 0.014923095703125, 0.00830078125, 0.005096435546875, 0.008941650390625, 0.01416015625, 0.01220703125, 0.0140380859375, 0.01275634765625, 0.006439208984375, 0.007049560546875, 0.006134033203125, -0.000457763671875, 0.003326416015625, 0.0081787109375, 0.009124755859375, 0.013458251953125, 0.014007568359375, 0.014312744140625, 0.006011962890625, 0.00238037109375, 0.010284423828125, 0.011962890625, 0.009857177734375, 0.00909423828125, 0.016448974609375, 0.01885986328125, 0.01190185546875, 0.010955810546875, 0.01019287109375, 0.00152587890625, 0.00762939453125, 0.008270263671875, 0.00604248046875, 0.010589599609375, 0.0037841796875, 0.0050048828125, 0.007080078125, 0.004669189453125, 0.0064697265625, 0.01068115234375, 0.009521484375, 0.002532958984375, -0.000518798828125, 0.005035400390625, 0.0042724609375, 0.00164794921875, 0.0001220703125, -0.002716064453125, -0.00164794921875, -0.007232666015625, -0.01153564453125, -0.005889892578125, -0.00341796875, -0.008514404296875, -0.007415771484375, -0.00726318359375, -0.007781982421875, -0.009918212890625, -0.010772705078125, -0.00628662109375, -0.001373291015625, -0.0008544921875, -0.003997802734375, 0.003021240234375, 0.003082275390625, 0.000640869140625, 0.00250244140625, 0.002960205078125, 0.00115966796875, 0.000579833984375, -0.002166748046875, -0.00115966796875, -0.006591796875, -0.0128173828125, -0.013275146484375, -0.0157470703125, -0.016204833984375, -0.013885498046875, -0.01531982421875, -0.00897216796875, -0.00762939453125, -0.00738525390625, -0.00311279296875, -0.002166748046875, 0.000244140625, -0.003509521484375, -0.003662109375, 0.001220703125, 0.001251220703125, 0.0001220703125, -0.003692626953125, -0.003997802734375, -0.004364013671875, -9.1552734375e-05, 0.00341796875, 0.000457763671875, -0.000274658203125, -0.0006103515625, 0.00543212890625, 0.001312255859375, 0.003662109375, 0.009765625, 0.004852294921875, 0.003997802734375, 0.00189208984375, -0.000213623046875, -0.006500244140625, -0.006744384765625, -0.0120849609375, -0.012359619140625, -0.003631591796875, -0.005645751953125, -0.0028076171875, 0.00286865234375, -0.00311279296875, -0.005279541015625, 0.001922607421875, -0.003753662109375, -0.000335693359375, -0.00299072265625, 0.001556396484375, 0.00299072265625, 0.006317138671875, 0.006622314453125, -0.003692626953125, -0.007110595703125, 0.001190185546875, -0.002288818359375, 0.00030517578125, 0.007720947265625, 0.003692626953125, 0.006011962890625, 0.007904052734375, 0.0115966796875, 0.01513671875, 0.00421142578125, 0.00299072265625, 0.002532958984375, 0.0009765625, 0.0018310546875, 0.001556396484375, 0.00640869140625, 0.008148193359375, 0.011962890625, 0.01416015625, 0.01055908203125, 0.0126953125, 0.006500244140625, 0.00958251953125, 0.009613037109375, 0.00921630859375, 0.007049560546875, 0.00927734375, 0.011871337890625, 0.015655517578125, 0.0146484375, 0.011627197265625, 0.0162353515625, 0.007965087890625, 0.00146484375, 0.004425048828125, 0.007415771484375, 0.007598876953125, 0.011810302734375, 0.01324462890625, 0.016357421875, 0.0126953125, 0.012451171875, 0.01763916015625, 0.0196533203125, 0.019775390625, 0.021453857421875, 0.025848388671875, 0.023468017578125, 0.01934814453125, 0.019073486328125, 0.020355224609375, 0.021270751953125, 0.024139404296875, 0.02545166015625, 0.0255126953125, 0.027862548828125, 0.027435302734375, 0.030487060546875, 0.029052734375, 0.032196044921875, 0.030120849609375, 0.035552978515625, 0.026611328125, 0.025787353515625, 0.030303955078125, 0.021270751953125, 0.027099609375, 0.032379150390625, 0.03143310546875, 0.02508544921875, 0.03118896484375, 0.029510498046875, 0.0311279296875, 0.03460693359375, 0.0340576171875, 0.027435302734375, 0.03076171875, 0.031707763671875, 0.029815673828125, 0.0341796875, 0.039337158203125, 0.0396728515625, 0.039459228515625, 0.031463623046875, 0.025482177734375, 0.03057861328125, 0.031707763671875, 
